vi "TreePath_to_XMLAttributePath.vi"(8 "error in (no error)":errorcluster, 10 "Tree Refnum":refnum<vi>, 11 "Tree Path (Array)":string[](array[string])) -> (0 "error out":errorcluster, 2 "XML Text Path (String)":string, 3 "XML Attribute path (String)":string)   [LabVIEW 2012]
doc: "SciScan 1.2 160622"
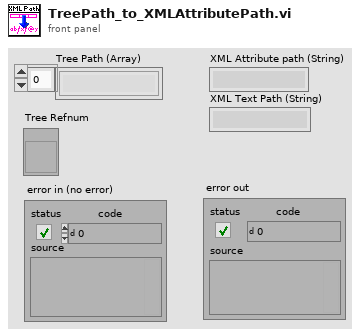
[diagram p1: front panel]
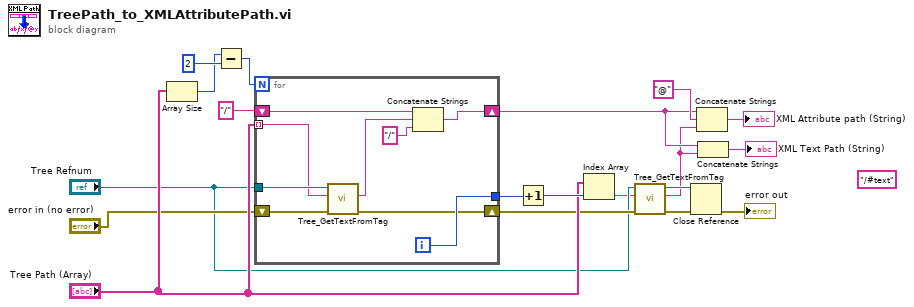
[diagram p0: block diagram]
diagram:
  (unwired) "/#text" ("string")
  n1 = Array Size(array="Tree Path (Array)") -> (size(s)=w11:i32)
  n2 = Subtract(x=w11, y=2 ("length")) -> (x-y=w13:i32)
  n3 = for {
    N: w13 -> [_]
    tunnel: "Tree Path (Array)" -> [w23] mode=indexing
    shift-right: [w28] -> w3
    shift-left: "/" ("string") -> [w26]
    tunnel: [w25] -> w15
    tunnel: "Tree Refnum" -> [w24]
    shift-right: [w20] -> w9
    shift-left: "error in (no error)" -> [w21]
    i -> [w25]
    n4 = call "Tree_GetTextFromTag.vi"("Error In"=w21, "Tag IN"=w23, "Tree Refnum IN"=w24) -> ("Error Out"=w20:errorcluster, "String OUT"=w22:string)  [unwired: 6 in, 1 out]
    n5 = Concatenate Strings(w26, w22, "/" ("string")) -> (w28:string)
  }
  n6 = Increment(x=w15) -> (x+1=w18:i32)
  n7 = Index Array(array="Tree Path (Array)", index=w18) -> (element=w7:string)
  n8 = call "Tree_GetTextFromTag.vi"("Error In"=w9, "Tag IN"=w7, "Tree Refnum IN"="Tree Refnum") -> ("Error Out"=w6:errorcluster, "String OUT"=w2:string, "Tree Refnum OUT"=w5:refnum<vi>)  [unwired: 6 in]
  n9 = Close Reference(reference=w5, error in (no error)=w6) -> (error out=→"error out":errorcluster)
  n10 = Concatenate Strings(w3, "@" ("string"), w2) -> (→"XML Attribute path (String)":string)
  n11 = Concatenate Strings(w3, w2) -> (→"XML Text Path (String)":string)
